vi "单独插入10站（101&102数据）vi.vi"() -> ()   [LabVIEW 2014]
uses:
  <vilib>/addons/database/Connection.llb/DB Tools Open Connec (String).vi
  <vilib>/addons/database/NI_Database_API.lvlib
panel:
  in  "Oline日期":string="2021-04-19_11:09"
  in  "QRcode":string="20210419A0170"
  in  "插入 101—102数据____单个":bool
  out "数据":string[][](array[string])
  in  "路径":path
  in  "读取文件表格":bool
  in  "插入 101—102数据__批量":bool
  in  "停止":bool
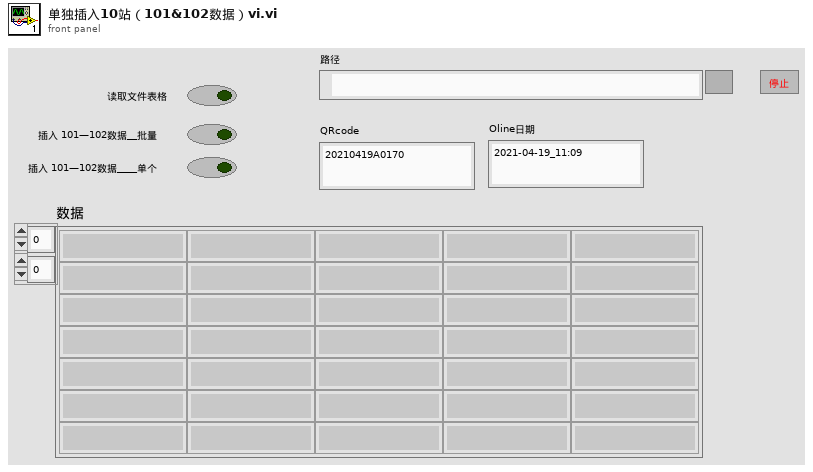
[diagram p1: front panel]
types:
  T1 = typedef "NI_Database_API.lvlib/Conn ObjectReference.ctl" = refnum<k1>
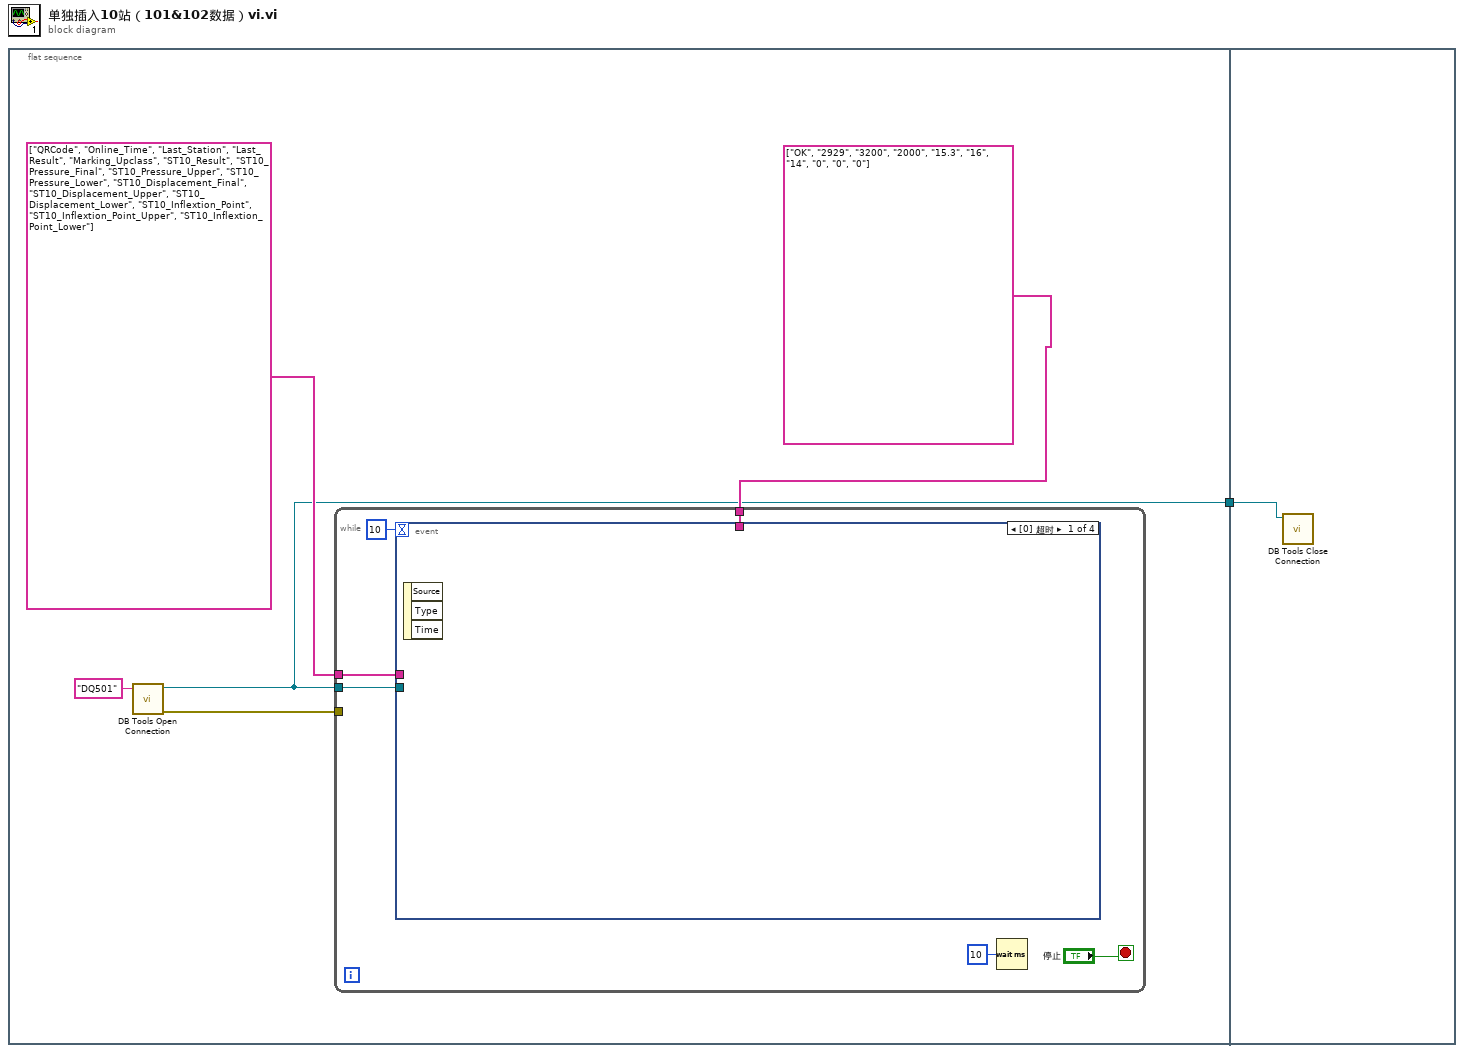
[diagram p0: block diagram]
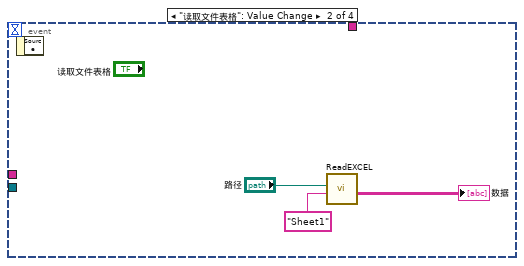
[diagram p2: hidden frame]
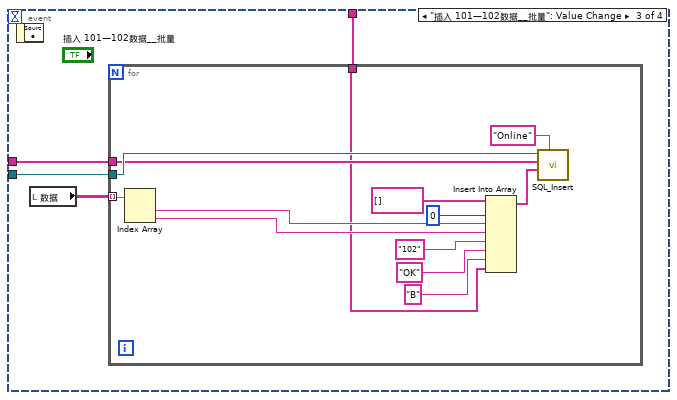
[diagram p3: hidden frame]
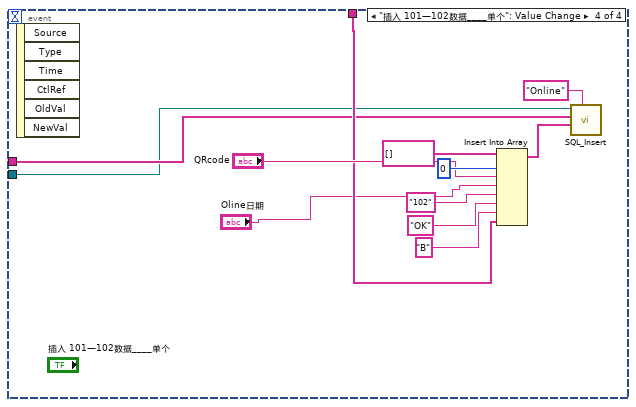
[diagram p4: hidden frame]
diagram:
  n1 = flat-sequence {
    tunnel: [w2] -> w1
    tunnel: w1 -> [w45]
    frame #0 {
      n2 = call-poly <vilib>:"DB Tools Open Connection.vi"("connection information"="DQ501") -> ("error out"=w5:errorcluster, "connection reference"=w2:T1)  [unwired: 7 in]
      n3 = while {
        tunnel: w2 -> [w9]
        tunnel: w5 -> [_]
        tunnel: string[] ["OK", "2929", "3200", "2000", "15.3", "16", "14", "0", "0", "0"] -> [w8]
        tunnel: string[] ["QRCode", "Online_Time", "Last_Station", "Last_Result", "Marking_Upclass", "ST10_Result", "ST10_Pressure_Final", "ST10_Pressure_Upper", "ST10_Pressure_Lower", "ST10_Displacement_Final", "ST10_Displacement_Upper", "ST10_Displacement_Lower", "ST10_Inflextion_Point", "ST10_Inflextion_Point_Upper", "ST10_Inflextion_Point_Lower"] ("列名") -> [w7]
        stop <- "停止" stop-if-true
        n4 = event shown="[0] 超时" {
          selector: _ -> [_ _ _ _]
          dyn-events: _ -> [_ _ _ _]
          timeout: 10 -> [_ _ _ _]
          tunnel: w9 -> [_ _ w18 w34]
          tunnel: w8 -> [_ _ w17 w36]
          tunnel: w7 -> [_ _ w16 w35]
          event Timeout {
            n5 = event-data() -> ()  [unwired: 1 in, 3 out]
          }
          event "读取文件表格": Value Change {
            n6 = event-data() -> ()  [unwired: 1 in, 1 out]
            n7 = call "ReadEXCEL.vi"("EXCEL 标签"="Sheet1", "路径"="路径") -> ("数据"=→"数据":string[][])  [unwired: 8 in, 1 out]
          }
          event "插入 101—102数据__批量": Value Change {
            n8 = event-data() -> ()  [unwired: 1 in, 1 out]
            n9 = local read "数据"() -> (w19:string[][])
            n10 = for {
              tunnel: w19 -> [w32] mode=indexing
              tunnel: w18 -> [w25]
              tunnel: w17 -> [w20]
              tunnel: w16 -> [w21]
              n11 = Index Array(array=w32) -> (element #1=w24:string, element #2=w23:string)  [unwired: 2 in]
              n12 = Insert Into Array(array=string[] [] ("数组"), index=0 ("索引"), new element #1=w24, new element #2=w23, new element #3="102" ("新元素/子数组"), new element #4="OK" ("新元素/子数组"), new element #5="B" ("新元素/子数组"), new element #6=w20) -> (w29:string[])
              n13 = call "SQL_Insert.vi"("表名"="Online", "值"=w29, "列名"=w21, "connection reference"=w25) -> ()  [unwired: 6 in, 2 out]
            }
          }
          event "插入 101—102数据____单个": Value Change {
            n14 = event-data() -> ()  [unwired: 1 in, 6 out]
            n15 = Insert Into Array(array=string[] [] ("数组"), index=0 ("索引"), new element #1="QRcode", new element #2="Oline日期", new element #3="102" ("新元素/子数组"), new element #4="OK" ("新元素/子数组"), new element #5="B" ("新元素/子数组"), new element #6=w36) -> (w42:string[])
            n16 = call "SQL_Insert.vi"("表名"="Online", "值"=w42, "列名"=w35, "connection reference"=w34) -> ()  [unwired: 6 in, 2 out]
          }
        }
        n17 = Wait (ms)(milliseconds to wait=u32 10 ("等待时间（毫秒）")) -> ()  [unwired: 1 out]
      }
    }
    frame #1 {
      n18 = call <vilib>:"DB Tools Close Connection.vi"("connection reference"=w45) -> ()  [unwired: 6 in, 1 out]
    }
  }
